vi "Close rotary stage.vi"(8 "error in (no error)":errorcluster, 11 "AOTF in":refnum<class "AOTF.lvclass">) -> (0 "error out":errorcluster, 3 "AOTF out":refnum<class "AOTF.lvclass">)   [LabVIEW 2012, in "AOTF.lvclass"]
uses:
  AOTF.lvclass
  AOTF.lvclass/AOTF.ctl
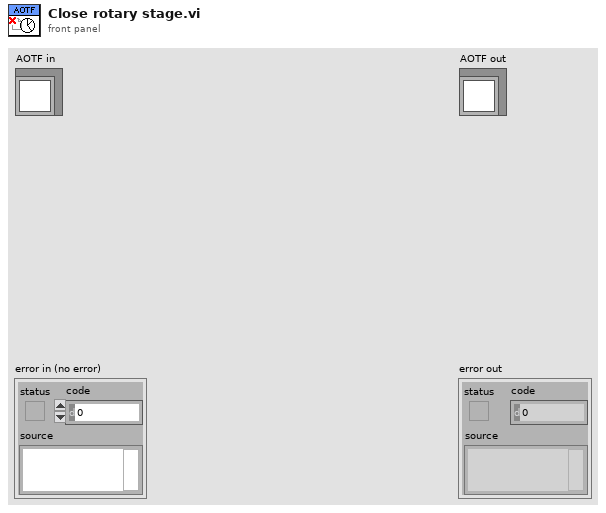
[diagram p1: front panel]
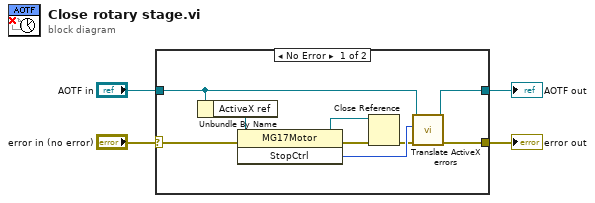
[diagram p0: block diagram]
diagram:
  n1 = case shown="No Error" "error in (no error)" {
    selector: "error in (no error)" -> [w8 w15]
    tunnel: [w5 w15] -> w3
    tunnel: [w6 w14] -> w1
    tunnel: "AOTF in" -> [w7 w14]
    frame No Error {
      n2 = Unbundle By Name(w7) -> ("ActiveX ref"=w13:refnum<k7>)
      n3 = invoke class="MG17Motor" method="StopCtrl"(reference=w13, error in=w8) -> (reference out=w11:refnum<k7>, error out=w10:errorcluster, "StopCtrl"=w12:i32)  [unwired: 1 in]
      n4 = Close Reference(reference=w11, error in (no error)=w10) -> (error out=w9:errorcluster)
      n5 = call-dynamic "Translate ActiveX errors.vi"("error in (no error)"=w9, "ActiveX return"=w12, "AOTF in"=w7) -> ("error out"=w5:errorcluster, "AOTF out"=w6:refnum<class "AOTF.lvclass">)  [unwired: 7 in]
    }
    frame Error {
    }
  }
  "error out" <- w3
  "AOTF out" <- w1
